vi "ADI_IMU_ADIS16448_Open.vi"(5 "Calibrate On Open":bool=TRUE, 7 "Calibration Time (s)":dbl=3.0, 8 "error in":errorcluster, 9 "AHRS Algorithm":enum16{"Complementary", "Madgwick"}(ring), 10 "Yaw Axis":enum16{"X", "Y", "Z"}(ring)=enum."Z", 11 "SPI Chip Select":T2=enum."SPI MXP") -> (0 "error out":errorcluster, 2 "Offset Compensated Data Out":dbl[](array[numeric]), 3 "ADI IMU DevRef Out":T1={"DevStatus"={"status"=FALSE, "code"=0, "source"=""}, "Handle"=0, "SPI Bus"=enum."SPI On-Board, CS0", "Device Found"=FALSE, "Device Ready"=FALSE, "Yaw Axis"=enum."Z", "AHRS Algorithm"=enum."Complementary", "Serial"=0, "Lot ID 2"=0, "Lot ID 1"=0, "Bytes Per Sample"=0, "Calibrate On Open?"=FALSE})   [LabVIEW 2017, in "ADIS16448_IMU.lvlib"]
doc: "Initiates communication between an Analog Devices MXP IMU and the RoboRIO."
uses:
  ADIS16448_IMU.lvlib
  <vilib>/Rock Robotics/SystemInterfaces/spilib/spi_bus.ctl
  ADI_IMU_ADIS16448_IMUDevRef.ctl
  <vilib>/Rock Robotics/WPI/SPI/WPI_SPIMode.ctl
  <vilib>/Rock Robotics/SystemInterfaces/DIO/FPGA_DIOChannel.ctl
  ADI_IMU_ADIS16448_Registers.ctl
  <vilib>/Rock Robotics/SystemInterfaces/NetworkCommunication/NetComm_UsageReport_ResourceType.ctl
  <vilib>/Rock Robotics/WPI/Counter/WPI_CounterDigitalInputToDigitalSource.vi
  ADI_IMU_ADIS16448_Loop.vi
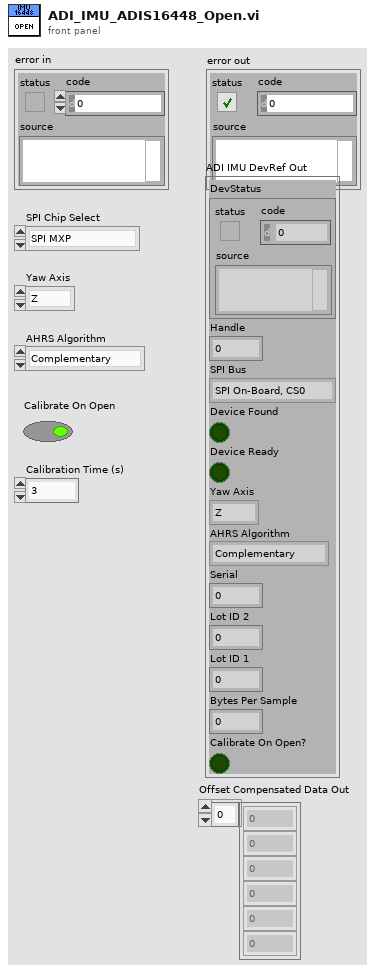
[diagram p1: front panel]
types:
  T1 = typedef "ADIS16448_IMU.lvlib/ADI_IMU_ADIS16448_IMUDevRef.ctl" = cluster{"DevStatus":errorcluster, "Handle":i32, "SPI Bus":T2, "Device Found":bool, "Device Ready":bool, "Yaw Axis":enum16{"X", "Y", "Z"}, "AHRS Algorithm":enum16{"Complementary", "Madgwick"}, "Serial":u16, "Lot ID 2":u16, "Lot ID 1":u16, "Bytes Per Sample":u16, "Calibrate On Open?":bool}
  T2 = typedef "spi_bus.ctl" = enum16{"SPI On-Board, CS0", "SPI On-Board, CS1", "SPI On-Board, CS2", "SPI On-Board, CS3", "SPI MXP", "Invalid"}
  T3 = typedef "FPGA_DIOChannel.ctl" = enum8{"DIO 0", "DIO 1", "DIO 2", "DIO 3", "DIO 4", "DIO 5", "DIO 6", "DIO 7", "DIO 8", "DIO 9", "DIO MXP 0", "DIO MXP 1", "DIO MXP 2", "DIO MXP 3", "DIO MXP 4", "DIO MXP 5", "DIO MXP 6", "DIO MXP 7", "DIO MXP 8", "DIO MXP 9", "DIO MXP 10", "DIO MXP 11", "DIO MXP 12", "DIO MXP 13", "DIO MXP 14", "DIO MXP 15", "SPI Port CS1", "SPI Port CS2", "SPI Port CS3", "SPI Port MISO", "SPI Port MOSI", "Invalid"}
  T4 = typedef "WPI_SPIMode.ctl" = enum16{"Mode 0 (Clk Idle Low,Sample on Leading)", "Mode 1 (Clk Idle Low,Sample on Trailing)", "Mode 2 (Clk Idle High,Sample on Leading)", "Mode 3 (Clk Idle High,Sample on Trailing)"}
  T5 = typedef "NetComm_UsageReport_ResourceType.ctl" = enum8{"Controller", "Module", "Language", "CANPlugin", "Accelerometer", "ADXL345", "AnalogChannel", "AnalogTrigger", "AnalogTriggerOutput", "CANJaguar", "Compressor", "Counter", "Dashboard", "DigitalInput", "DigitalOutput", "DriverStationCIO", "DriverStationEIO", "DriverStationLCD", "Encoder", "GearTooth", "Gyro", "I2C", "Framework", "Jaguar", "Joystick", "Kinect", "KinectStick", "PIDController", "Preferences", "PWM", "Relay", "RobotDrive", "SerialPort", "Servo", "Solenoid", "SPI", "Task", "Ultrasonic", "Victor", "Button", "Command", "AxisCamera", "PCVideoServer", "SmartDashboard", "Talon", "HiTechnicColorSensor", "HiTechnicAccel", "HiTechnicCompass", "SRF08", "AnalogOutput", "Victor SP", "Talon SRX", "CAN Talon SRX", "ADXL362 Accel", "ADXRS450 Gyro", "Rev SPARK", "Mindsensors SD540", "Digital Filter", "ADIS16448", "PDP", "PCM", "PigeonIMU", "Nidec Brushless", "CTRE CANifier", "CTRE Future 0", "CTRE Future 1", "CTRE Future 2", "CTRE Future 3", "CTRE Future 4", "CTRE Future 5", "CTRE Future 6"}
  T6 = typedef "ADIS16448_IMU.lvlib/ADI_IMU_ADIS16448_Registers.ctl" = u8
  T7 = typedef "WPI_DigitalOutputDevRef.ctl" = cluster{"DIO Channel":T3, "DevStatus":errorcluster}
  T8 = typedef "WPI_DigitalInputDevRef.ctl" = cluster{"DevStatus":errorcluster, "DIO Channel":T3}
  T9 = typedef "WPI_SPIDevRef.ctl" = cluster{"DevStatus":errorcluster, "Handle":i32, "SPI Bus":T2}
  T10 = typedef "FPGA_CounterEncoderSourceConvertionLVSourceType.ctl" = cluster{"DevStatus":errorcluster, "AnalogTriggerMode?":bool, "DigitalMode":cluster{"DIO Channel":T11}, "AnalogTriggerMode":cluster{"AnalogTriggerIndex":T12, "OutputType":T13}}
  T11 = typedef "FPGA_DIODigitalSourceChannel.ctl" = enum8{"DIO 0", "DIO 1", "DIO 2", "DIO 3", "DIO 4", "DIO 5", "DIO 6", "DIO 7", "DIO 8", "DIO 9", "DIO MXP 0", "DIO MXP 1", "DIO MXP 2", "DIO MXP 3", "DIO MXP 4", "DIO MXP 5", "DIO MXP 6", "DIO MXP 7", "DIO MXP 8", "DIO MXP 9", "DIO MXP 10", "DIO MXP 11", "DIO MXP 12", "DIO MXP 13", "DIO MXP 14", "DIO MXP 15", "Disabled"}
  T12 = typedef "FPGA_AnalogTriggerIndex.ctl" = enum8{"Trig 0", "Trig 1", "Trig 2", "Trig 3", "Trig 4", "Trig 5", "Trig 6", "Trig 7", "Invalid"}
  T13 = typedef "FPGA_AnalogTriggerOutType.ctl" = enum16{"InWindow", "TriggerState", "Rising", "Falling"}
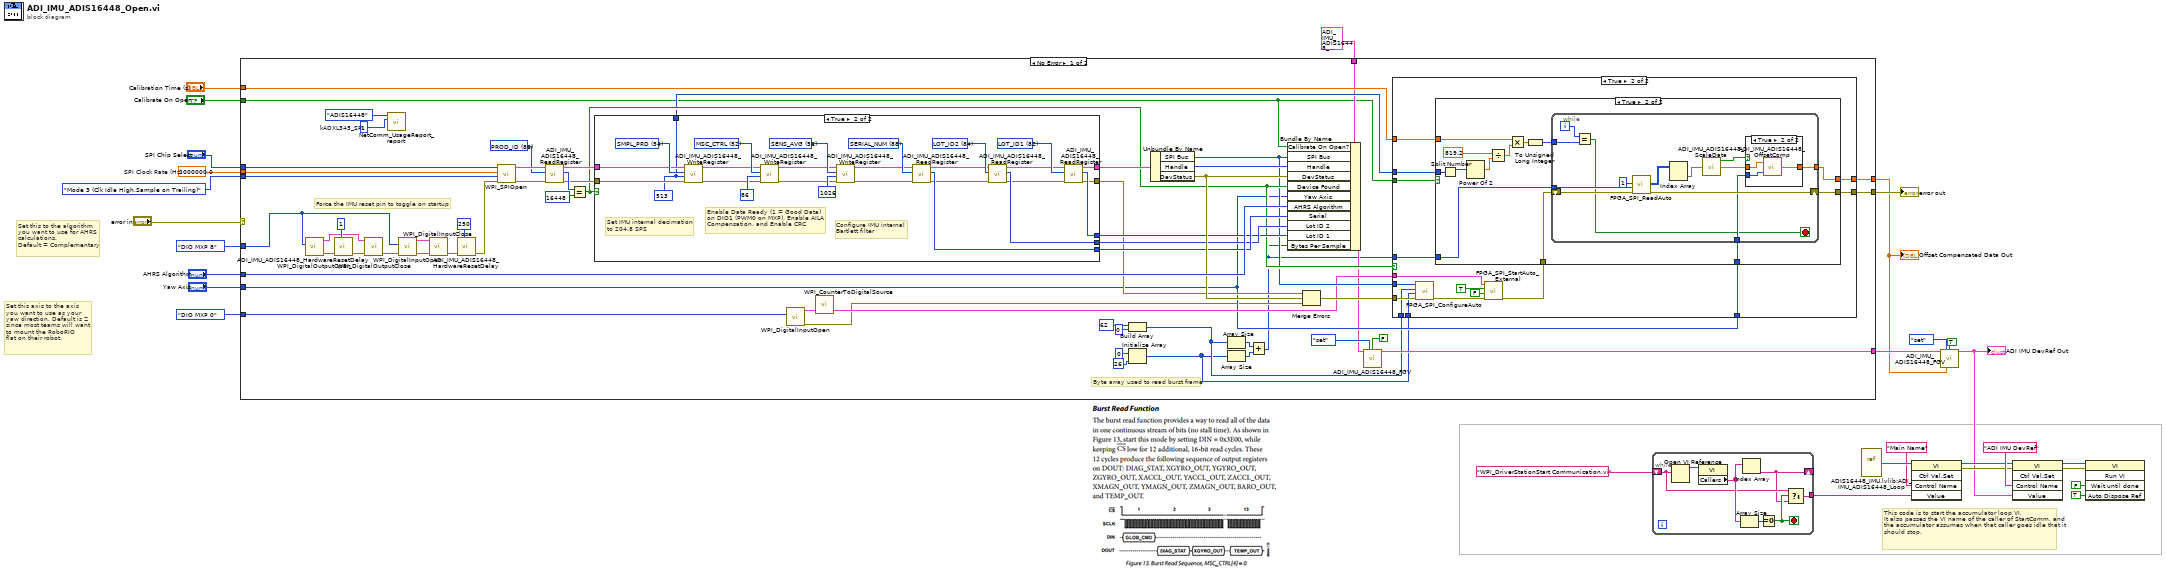
[diagram p0: block diagram]
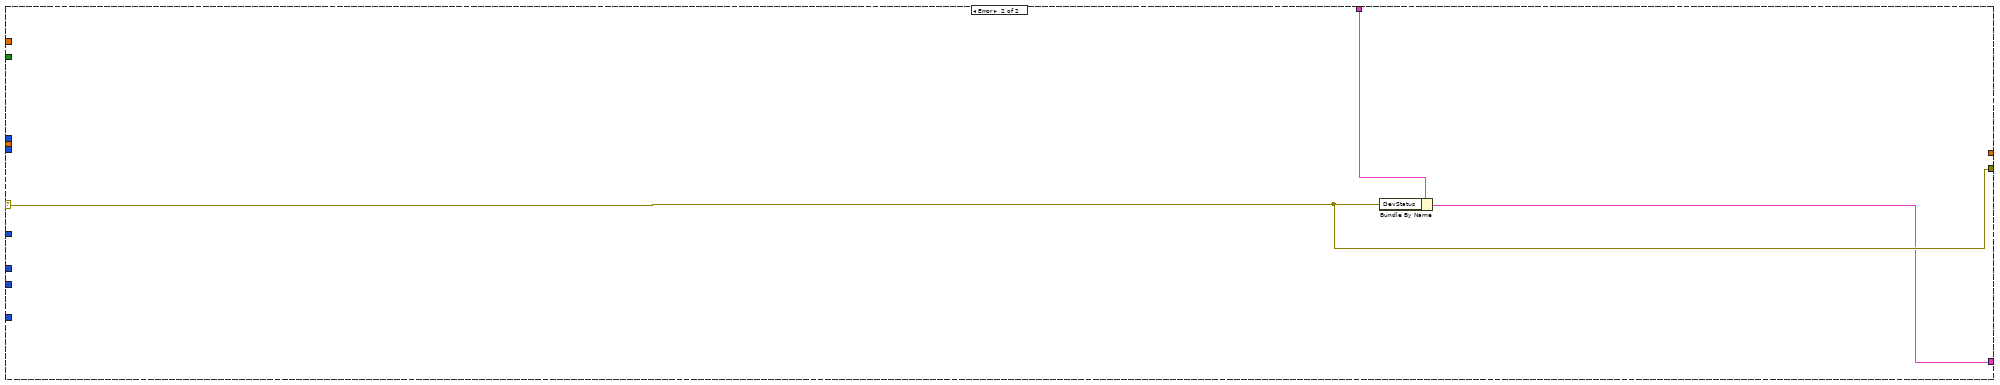
[diagram p6: hidden frame]
diagram:
  w28 = 1000000.0  # SPI Clock Rate (Hz)
  # "This code is to start the accumulator loop VI.\nIt also passes the VI name of the caller of StartComm, and the accumulator assumes when that caller goes idle that it should stop."
  # "Set this to the algorithm\nyou want to use for AHRS\ncalculations. \nDefault = Complementary"
  # "Set this axis to the axis\nyou want to use as your\nyaw direction. Default is Z\nsince most teams will want \nto mount the RoboRIO\nflat on their robot."
  n1 = case shown="No Error" "error in" {
    selector: "error in" -> [_ w164]
    tunnel: w28 -> [w86 _]
    tunnel: WPI_SPIMode."Mode 3 (Clk Idle High,Sample on Trailing)" ("Mode (3)") -> [w85 _]
    tunnel: "SPI Chip Select" -> [w84 _]
    tunnel: FPGA_DIOChannel."DIO MXP 0" ("DIO Channel") -> [w61 _]
    tunnel: "Yaw Axis" -> [w56 _]
    tunnel: "AHRS Algorithm" -> [w83 _]
    tunnel: FPGA_DIOChannel."DIO MXP 8" ("DIO Channel") -> [w82 _]
    tunnel: "Calibrate On Open" -> [w29 _]
    tunnel: "Calibration Time (s)" -> [w57 _]
    tunnel: T1 {"DevStatus"={"status"=FALSE, "code"=0, "source"=""}, "Handle"=0, "SPI Bus"=enum."SPI On-Board, CS0", "Device Found"=FALSE, "Device Ready"=FALSE, "Yaw Axis"=enum."Z", "AHRS Algorithm"=enum."Complementary", "Serial"=0, "Lot ID 2"=0, "Lot ID 1"=0, "Bytes Per Sample"=0, "Calibrate On Open?"=FALSE} ("SimpleGyroDevRef 2") -> [w55 w165]
    tunnel: [w54 w164] -> w6
    tunnel: [w50 w163] -> w3
    tunnel: [w49 _] -> w2
    frame No Error {
      w75 = u8 1  # kADXL345_SPI
      w71 = T6 86 items=["GLOB_CMD"=62, "SEQ_CNT"=58, "SMPL_PRD"=54, "SENS_AVG"=56, "MSC_CTRL"=52, "ERROR_FLAGS"=60, "TEMP"=44, "BARO"=40, "Z_MAG"=36, "Y_MAG"=32, "X_MAG"=28, "Z_ACCEL"=24, "Y_ACCEL"=20, "X_ACCEL"=16, "Z_GYRO"=12, "Y_GYRO"=8, "X_GYRO"=4, "PROD_ID"=86, "LOT_ID2"=84, "LOT_ID1"=82, "SERIAL_NUM"=88] ("ADIS16448 Register")
      # "Byte array used to read burst frame"
      # "Force the IMU reset pin to toggle on startup"
      n2 = call <vilib>:"WPI_DigitalOutputOpen.vi"("DIO Channel"=w82) -> ("error out"=w46:errorcluster, "DigitalOutputDevRef"=w40:T7)  [unwired: 9 in]
      n3 = call "ADI_IMU_ADIS16448_HardwareResetDelay.vi"("Delay (ms)"=u32 1, "error in"=w46) -> ("error out"=w47:errorcluster)  [unwired: 9 in]
      n4 = call <vilib>:"WPI_DigitalOutputClose.vi"("error in (no error)"=w47, "DigitalOutputDevRef"=w40) -> ("error out"=w45:errorcluster)  [unwired: 9 in]
      n5 = call <vilib>:"NetComm_UsageReport_report.vi"("Instance Number"=w75, "Resource Type"=NetComm_UsageReport_ResourceType."ADIS16448") -> ()  [unwired: 10 in]
      n6 = call <vilib>:"WPI_DigitalInputOpen.vi"("error in (no error)"=w45, "DIO Channel"=w82) -> ("error out"=w44:errorcluster, "DigitalInputDevRef"=w43:T8)  [unwired: 8 in]
      n7 = call <vilib>:"WPI_DigitalInputClose.vi"("error in (no error)"=w44, "DigitalInputDevRef"=w43) -> ("error out"=w42:errorcluster)  [unwired: 9 in]
      n8 = call "ADI_IMU_ADIS16448_HardwareResetDelay.vi"("Delay (ms)"=u32 250, "error in"=w42) -> ("error out"=w76:errorcluster)  [unwired: 9 in]
      n9 = call <vilib>:"WPI_SPIOpen.vi"("error in"=w76, "Mode (3)"=w85, "Clock Rate (Hz)"=w86, "SPI Bus"=w84) -> ("error out"=w72:errorcluster, "SPIDevRef"=w73:T9)  [unwired: 6 in]
      n10 = call "ADI_IMU_ADIS16448_ReadRegister.vi"("error in (no error)"=w72, "ADIS16448 Register"=w71, "SPIDevRef in"=w73) -> ("error out"=w67:errorcluster, "Register Value"=w70:u16, "SPIDevRef out"=w68:T9)  [unwired: 6 in]
      n11 = Equal?(x=w70, y=u16 16448) -> (x = y?=w63:bool)
      n12 = case shown="True" w63 {
        tunnel: [_ w156] -> w79
        tunnel: [_ w155] -> w78
        tunnel: [_ w153] -> w77
        tunnel: [w136 w141] -> w66
        tunnel: [w135 w140] -> w65
        tunnel: w68 -> [w136 w139]
        tunnel: w67 -> [w135 w138]
        tunnel: [_ w137] -> w58
        frame False {
        }
        frame True {
          w152 = T6 82 items=["GLOB_CMD"=62, "SEQ_CNT"=58, "SMPL_PRD"=54, "SENS_AVG"=56, "MSC_CTRL"=52, "ERROR_FLAGS"=60, "TEMP"=44, "BARO"=40, "Z_MAG"=36, "Y_MAG"=32, "X_MAG"=28, "Z_ACCEL"=24, "Y_ACCEL"=20, "X_ACCEL"=16, "Z_GYRO"=12, "Y_GYRO"=8, "X_GYRO"=4, "PROD_ID"=86, "LOT_ID2"=84, "LOT_ID1"=82, "SERIAL_NUM"=88] ("ADIS16448 Register")
          w154 = T6 84 items=["GLOB_CMD"=62, "SEQ_CNT"=58, "SMPL_PRD"=54, "SENS_AVG"=56, "MSC_CTRL"=52, "ERROR_FLAGS"=60, "TEMP"=44, "BARO"=40, "Z_MAG"=36, "Y_MAG"=32, "X_MAG"=28, "Z_ACCEL"=24, "Y_ACCEL"=20, "X_ACCEL"=16, "Z_GYRO"=12, "Y_GYRO"=8, "X_GYRO"=4, "PROD_ID"=86, "LOT_ID2"=84, "LOT_ID1"=82, "SERIAL_NUM"=88] ("ADIS16448 Register")
          w157 = T6 88 items=["GLOB_CMD"=62, "SEQ_CNT"=58, "SMPL_PRD"=54, "SENS_AVG"=56, "MSC_CTRL"=52, "ERROR_FLAGS"=60, "TEMP"=44, "BARO"=40, "Z_MAG"=36, "Y_MAG"=32, "X_MAG"=28, "Z_ACCEL"=24, "Y_ACCEL"=20, "X_ACCEL"=16, "Z_GYRO"=12, "Y_GYRO"=8, "X_GYRO"=4, "PROD_ID"=86, "LOT_ID2"=84, "LOT_ID1"=82, "SERIAL_NUM"=88] ("ADIS16448 Register")
          w158 = T6 56 items=["GLOB_CMD"=62, "SEQ_CNT"=58, "SMPL_PRD"=54, "SENS_AVG"=56, "MSC_CTRL"=52, "ERROR_FLAGS"=60, "TEMP"=44, "BARO"=40, "Z_MAG"=36, "Y_MAG"=32, "X_MAG"=28, "Z_ACCEL"=24, "Y_ACCEL"=20, "X_ACCEL"=16, "Z_GYRO"=12, "Y_GYRO"=8, "X_GYRO"=4, "PROD_ID"=86, "LOT_ID2"=84, "LOT_ID1"=82, "SERIAL_NUM"=88] ("ADIS16448 Register")
          w159 = T6 52 items=["GLOB_CMD"=62, "SEQ_CNT"=58, "SMPL_PRD"=54, "SENS_AVG"=56, "MSC_CTRL"=52, "ERROR_FLAGS"=60, "TEMP"=44, "BARO"=40, "Z_MAG"=36, "Y_MAG"=32, "X_MAG"=28, "Z_ACCEL"=24, "Y_ACCEL"=20, "X_ACCEL"=16, "Z_GYRO"=12, "Y_GYRO"=8, "X_GYRO"=4, "PROD_ID"=86, "LOT_ID2"=84, "LOT_ID1"=82, "SERIAL_NUM"=88] ("ADIS16448 Register")
          w160 = T6 54 items=["GLOB_CMD"=62, "SEQ_CNT"=58, "SMPL_PRD"=54, "SENS_AVG"=56, "MSC_CTRL"=52, "ERROR_FLAGS"=60, "TEMP"=44, "BARO"=40, "Z_MAG"=36, "Y_MAG"=32, "X_MAG"=28, "Z_ACCEL"=24, "Y_ACCEL"=20, "X_ACCEL"=16, "Z_GYRO"=12, "Y_GYRO"=8, "X_GYRO"=4, "PROD_ID"=86, "LOT_ID2"=84, "LOT_ID1"=82, "SERIAL_NUM"=88] ("ADIS16448 Register")
          w137 = u16 513 ("Data")
          # "Configure IMU internal\nBartlett filter"
          # "Enable Data Ready (1 = Good Data) \non DIO1 (PWM0 on MXP), Enable AILA\nCompensation, and Enable CRC"
          # "Set IMU internal decimation\nto 204.8 SPS"
          n13 = call "ADI_IMU_ADIS16448_WriteRegister.vi"("error in (no error)"=w138, "Data"=w137, "ADIS16448 Register"=w160, "SPIDevRef in"=w139) -> ("error out"=w150:errorcluster, "SPIDevRef out"=w151:T9)  [unwired: 6 in]
          n14 = call "ADI_IMU_ADIS16448_WriteRegister.vi"("error in (no error)"=w150, "Data"=u16 86, "ADIS16448 Register"=w159, "SPIDevRef in"=w151) -> ("error out"=w148:errorcluster, "SPIDevRef out"=w149:T9)  [unwired: 6 in]
          n15 = call "ADI_IMU_ADIS16448_WriteRegister.vi"("error in (no error)"=w148, "Data"=u16 1026, "ADIS16448 Register"=w158, "SPIDevRef in"=w149) -> ("error out"=w146:errorcluster, "SPIDevRef out"=w147:T9)  [unwired: 6 in]
          n16 = call "ADI_IMU_ADIS16448_ReadRegister.vi"("error in (no error)"=w146, "ADIS16448 Register"=w157, "SPIDevRef in"=w147) -> ("error out"=w144:errorcluster, "Register Value"=w156:u16, "SPIDevRef out"=w145:T9)  [unwired: 6 in]
          n17 = call "ADI_IMU_ADIS16448_ReadRegister.vi"("error in (no error)"=w144, "ADIS16448 Register"=w154, "SPIDevRef in"=w145) -> ("error out"=w142:errorcluster, "Register Value"=w155:u16, "SPIDevRef out"=w143:T9)  [unwired: 6 in]
          n18 = call "ADI_IMU_ADIS16448_ReadRegister.vi"("error in (no error)"=w142, "ADIS16448 Register"=w152, "SPIDevRef in"=w143) -> ("error out"=w140:errorcluster, "Register Value"=w153:u16, "SPIDevRef out"=w141:T9)  [unwired: 6 in]
        }
      }
      n19 = call <vilib>:"WPI_DigitalInputOpen.vi"("DIO Channel"=w61) -> ("error out"=w39:errorcluster, "DigitalInputDevRef"=w60:T8)  [unwired: 9 in]
      n20 = call-poly <vilib>:"WPI_CounterToDigitalSource.vi"("DigitalInputDevRef"=w60) -> ("Digital Source"=w59:T10)  [unwired: 6 in]
      n21 = Build Array(u8 62 ("hi"), u8 0 ("element")) -> (w32:u8[])
      n22 = Initialize Array(u8 0 ("element"), 26 ("dimension size")) -> (w31:u8[])
      n23 = Unbundle By Name(w66) -> ("SPI Bus"=w62:T2, "Handle"=w81:i32, "DevStatus"=w80:errorcluster)
      n24 = Array Size(array=w32) -> (size(s)=w34:i32)
      n25 = Array Size(array=w31) -> (size(s)=w33:i32)
      n26 = Add(x=w34, y=w33) -> (x+y=w30:i32)
      n27 = Bundle By Name(cluster=w55, "Calibrate On Open?"=w29, "SPI Bus"=w62, "Handle"=w81, "DevStatus"=w80, "Device Found"=w63, "Yaw Axis"=w56, "AHRS Algorithm"=w83, "Serial"=w79, "Lot ID 2"=w78, "Lot ID 1"=w77, "Bytes Per Sample"=w30) -> (w51:T1)
      n28 = Merge Errors(w65, w80, w39) -> (w64:errorcluster)
      n29 = call "ADI_IMU_ADIS16448_FGV.vi"("ADI IMU DevRef"=w51, "Operation"=enum16{"set", "get", "set reset"}."set", "Sensor Ready?"=FALSE) -> ("ADI IMU DevRef Out"=w50:T1)  [unwired: 6 in, 6 out]
      n30 = case shown="True" w63 {
        tunnel: w64 -> [w87 w103]
        tunnel: w62 -> [_ w102]
        tunnel: w32 -> [_ w90]
        tunnel: w59 -> [_ w98]
        tunnel: w29 -> [_ w97]
        tunnel: w58 -> [_ w95]
        tunnel: w57 -> [_ w94]
        tunnel: [_ w93] -> w49
        tunnel: w56 -> [_ w92]
        tunnel: [w87 w91] -> w54
        tunnel: w31 -> [_ w89]
        tunnel: w30 -> [_ w88]
        frame False {
        }
        frame True {
          n31 = call <vilib>:"FPGA_SPI_ConfigureAuto.vi"("SPI Bus"=w102, "SPI Auto TX Byte Array"=w90, "SPI Auto TX Zero Byte Array"=w89, "error in"=w103) -> ("error out"=w101:errorcluster)  [unwired: 6 in]
          n32 = call <vilib>:"FPGA_SPI_StartAuto_External.vi"("error in (no error)"=w101, "Falling Edge"=FALSE, "Rising Edge"=TRUE, "Source"=w98) -> ("error out"=w96:errorcluster)  [unwired: 7 in]
          n33 = case shown="True" w97 {
            tunnel: w96 -> [w104 w117]
            tunnel: w95 -> [_ w116]
            tunnel: w94 -> [_ w111]
            tunnel: [_ w109] -> w93
            tunnel: w92 -> [_ w110]
            tunnel: [w104 w108] -> w91
            tunnel: w88 -> [_ w105]
            frame False {
            }
            frame True {
              n34 = Split Number(x=w116) -> (hi(x)=w107:u8)  [unwired: 1 out]
              n35 = Power Of 2(x=w107) -> (2^x=w114:dbl)
              n36 = Divide(x=819.2, y=w114) -> (x/y=w113:dbl)
              n37 = Multiply(x=w111, y=w113) -> (x*y=w112:dbl)
              n38 = To Unsigned Long Integer(number=w112) -> (unsigned 32bit integer=w106:u32)
              n39 = while {
                shift-right: [w129] -> w108
                shift-left: w117 -> [w130]
                tunnel: w110 -> [w128]
                tunnel: [w127] -> w109
                tunnel: w105 -> [w125]
                tunnel: w106 -> [w122]
                i -> [w123]
                stop <- w121 stop-if-true
                n40 = Equal?(x=w123, y=w122) -> (x = y?=w121:bool)
                n41 = call <vilib>:"FPGA_SPI_ReadAuto.vi"("error in (no error)"=w130, "Bytes per Sample"=w125, "Samples to Read"=u32 1) -> ("error out"=w129:errorcluster, "Data"=w120:u8[][])  [unwired: 7 in]
                n42 = Index Array(array=w120) -> (element=w119:u8[])  [unwired: 2 in]
                n43 = call "ADI_IMU_ADIS16448_ScaleData.vi"("Received Data"=w119) -> ("Data Array"=w126:dbl[], "Data Good?"=w118:bool)  [unwired: 3 in]
                n44 = case shown="True" w118 {
                  tunnel: w128 -> [_ w134]
                  tunnel: [w131 w133] -> w127
                  tunnel: w126 -> [w131 w132]
                  frame False {
                  }
                  frame True {
                    n45 = call "ADI_IMU_ADIS16448_OffsetComp.vi"("Yaw Axis"=w134, "Raw Data"=w132) -> ("Offset Compensated Data"=w133:dbl[])
                  }
                }
              }
            }
          }
        }
      }
    }
    frame Error {
      n46 = Bundle By Name(cluster=w165, "DevStatus"=w164) -> (w163:T1)
    }
  }
  "error out" <- w6
  "Offset Compensated Data Out" <- w2
  n47 = while {
    shift-right: [w167] -> _
    shift-left: "WPI_DriverStationStart Communication.vi" -> [w168]
    tunnel: [w166] -> w12
    stop <- w169 stop-if-true
    n48 = Open VI Reference(vi path=w168) -> (vi reference=w172:refnum<vi>)  [unwired: 1 in, 5 out]
    n49 = property class="VI"(reference=w172) -> ("Callers"=w170:string[])  [unwired: 1 in, 2 out]
    n50 = Array Size(array=w170) -> (size(s)=w171:i32)
    n51 = Index Array(array=w170) -> (element=w167:string)  [unwired: 1 in]
    n52 = Equal To 0?(x=w171) -> (x = 0?=w169:bool)
    n53 = Select(t=w168, s=w169, f=w167) -> (s? t:f=w166:string)
  }
  n54 = vi-ref "ADIS16448_IMU.lvlib:ADI_IMU_ADIS16448_Loop.vi"() -> (w14:refnum<vi>)
  n55 = invoke class="VI" method="Ctrl Val.Set"(reference=w14, "Control Name"="Main Name", "Value"=w12) -> (reference out=w11:refnum<vi>, error out=w16:errorcluster)  [unwired: 2 in, 3 out]
  n56 = call "ADI_IMU_ADIS16448_FGV.vi"("ADI IMU DevRef"=w3, "Operation"=enum16{"set", "get", "set reset"}."set", "Sensor Ready?"=TRUE, "Offset Compensated Data"=w2) -> ("ADI IMU DevRef Out"=w1:T1)  [unwired: 5 in, 6 out]
  "ADI IMU DevRef Out" <- w1
  n57 = invoke class="VI" method="Ctrl Val.Set"(reference=w11, error in=w16, "Control Name"="ADI IMU DevRef", "Value"=w1) -> (reference out=w21:refnum<vi>, error out=w17:errorcluster)  [unwired: 1 in, 3 out]
  n58 = invoke class="VI" method="Run VI"(reference=w21, error in=w17, "Wait until done"=FALSE ("Wait Until Done"), "Auto Dispose Ref"=TRUE ("Auto Dispose Reference")) -> ()  [unwired: 1 in, 5 out]
